vi "PID (Set).vi"(6 "ISOBUS address":T3=-1 caption="ISOBUS address (-1)", 8 "error in":errorcluster, 10 "P Value":T1 {"D" min=0.0 max=299.9 step=0.1 format="%#.1f"; "I" min=0.0 max=199.9 step=0.1 format="%#.1f"; "P" min=0.0 max=199.9 step=0.1 format="%#.1f"}, 11 "Mercury Reference In":T5) -> (0 "error out":errorcluster, 2 "Response":T2, 3 "Mercury Reference Out":T5, 4 "Valid?":T4)   [LabVIEW 2016, in "Mercury iXX.lvlib" / "Control Loop.lvlib"]
doc: "Set the PID associated with control loop."
uses:
  Control Loop.lvlib
  Controls/Mercury Reference.ctl
  Controls/Comms Transport Layer.ctl
  Private/Controls/Query Dynamic Reference.ctl
  Controls/Is Valid LED.ctl
  Controls/ISOBus Address.ctl
  Controls/Response String.ctl
  Controls/PID cluster.ctl
  Private/Controls/Command Verbs.ctl
  Mercury iXX.lvlib
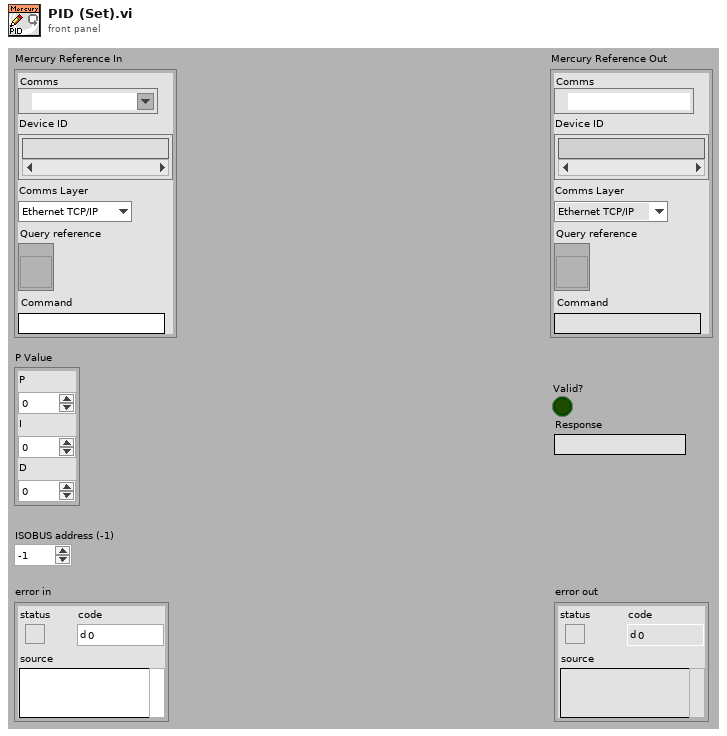
[diagram p1: front panel]
types:
  T1 = typedef "Mercury iXX.lvlib/Control Loop.lvlib/PID cluster.ctl" = cluster{"P":dbl, "I":dbl, "D":dbl}
  T2 = typedef "Mercury iXX.lvlib/Response String.ctl" = string
  T3 = typedef "Mercury iXX.lvlib/ISOBus Address.ctl" = i32
  T4 = typedef "Mercury iXX.lvlib/Is Valid LED.ctl" = bool
  T5 = typedef "Mercury iXX.lvlib/Mercury Reference.ctl" = cluster{"Comms":refnum<visa-resource-name>, "Device ID":string[], "Comms Layer":T6, "Command":string, "Query reference":T7}
  T6 = typedef "Mercury iXX.lvlib/Comms Transport Layer.ctl" = enum16{"Ethernet TCP/IP", "USB", "ISOBus - RS-232", "GPIB"}
  T7 = typedef "Mercury iXX.lvlib/Query Dynamic Reference.ctl" = refnum<vi>
  T8 = typedef "Mercury iXX.lvlib/Command Verbs.ctl" = string
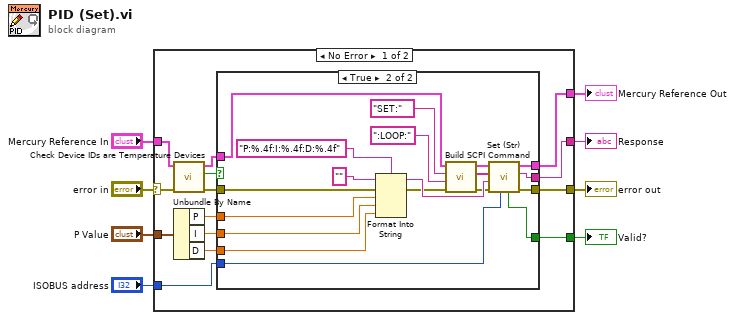
[diagram p0: block diagram]
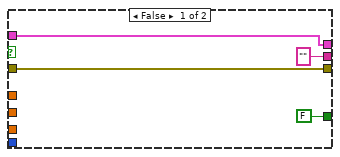
[diagram p2: hidden frame]
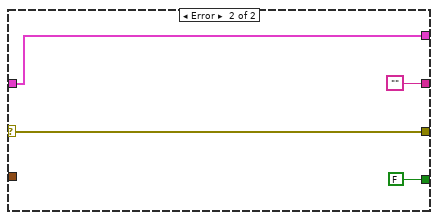
[diagram p3: hidden frame]
diagram:
  n1 = case shown="No Error" "error in" {
    selector: "error in" -> [w18 w48]
    tunnel: "Mercury Reference In" -> [w13 w49]
    tunnel: [w20 w49] -> w7
    tunnel: [w19 w48] -> w6
    tunnel: "ISOBUS address" -> [w21 _]
    tunnel: [w10 ""] -> w4
    tunnel: [w11 FALSE ("Valid?")] -> w5
    tunnel: "P Value" -> [w22 _]
    frame No Error {
      n2 = call "Check Device IDs are Temperature Devices.vi"("error in"=w18, "Mercury Reference In"=w13) -> ("error out"=w17:errorcluster, "Valid?"=w9:bool, "Mercury Reference Out"=w12:T5)  [unwired: 7 out]
      n3 = Unbundle By Name(w22) -> ("P"=w16:dbl, "I"=w15:dbl, "D"=w14:dbl)
      n4 = case shown="True" w9 {
        tunnel: w16 -> [_ w37]
        tunnel: w17 -> [w26 w34]
        tunnel: w21 -> [_ w27]
        tunnel: w12 -> [w25 w28]
        tunnel: [w25 w29] -> w20
        tunnel: [w26 w32] -> w19
        tunnel: w15 -> [_ w36]
        tunnel: w14 -> [_ w35]
        tunnel: [T4 FALSE ("Valid?") w31] -> w11
        tunnel: [T2 "" ("Response") w30] -> w10
        frame False {
        }
        frame True {
          n5 = Format Into String(format string="P:%.4f:I:%.4f:D:%.4f", initial string="", error in=w34, w37, w36, w35) -> (resulting string=w44:string, error out=w33:errorcluster)
          n6 = call "Build SCPI Command.vi"("error in"=w33, "Noun(s)"=":LOOP:", "Verb"=T8 "SET:", "Mercury Reference In"=w28) -> ("error out"=w41:errorcluster, "SCPI Message(s)"=w40:string[], "Mercury Reference Out"=w39:T5)  [unwired: 5 out]
          n7 = call "Set (Str).vi"("ISOBUS address"=w27, "error in"=w41, "Command Value (Str)"=w44, "SCPI Message(s)"=w40, "Mercury Reference In"=w39) -> ("error out"=w32:errorcluster, "Response"=w30:T2, "Mercury Reference Out"=w29:T5, "Valid?"=w31:T4)  [unwired: 3 out]
        }
      }
    }
    frame Error {
    }
  }
  "Mercury Reference Out" <- w7
  "error out" <- w6
  "Valid?" <- w5
  "Response" <- w4
